vi "Parse Motor Config Data.vi"(7 "Motor NO":u8, 8 "error in (no error)":errorcluster, 10 "PLC Data in":T1, 11 "Data Read":u8[][](array[numeric])) -> (0 "error out":errorcluster, 2 "PLC Data out":T1)   [LabVIEW 2018]
uses:
  Ctls/DisplayIndicator.ctl
  Ctls/MotroConfigData.ctl
  Ctls/MotorConfig.ctl
  Ctls/MagType.ctl
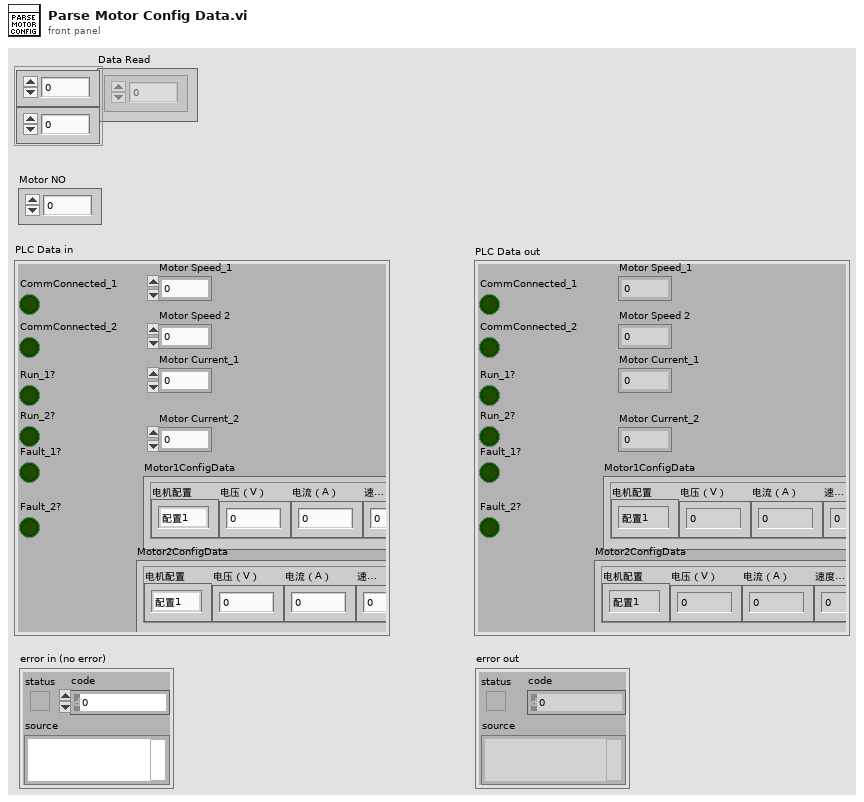
[diagram p1: front panel]
types:
  T1 = typedef "DisplayIndicator.ctl" = cluster{"CommConnected_1":bool, "Run_1?":bool, "Fault_1?":bool, "CommConnected_2":bool, "Run_2?":bool, "Fault_2?":bool, "Motor Speed 2":sgl, "Motor Speed_1":sgl, "Motor Current_1":sgl, "Motor Current_2":sgl, "Motor1ConfigData":T2, "Motor2ConfigData":T2}
  T2 = typedef "MotroConfigData.ctl" = cluster{"电机配置":T3, "电压（V）":dbl, "电流（A）":dbl, "速度（RPM）":dbl, "励磁方式":T4}
  T3 = typedef "MotorConfig.ctl" = enum16{"配置1", "配置2", "配置3", "配置4"}
  T4 = typedef "MagType.ctl" = enum16{"永磁", "励磁"}
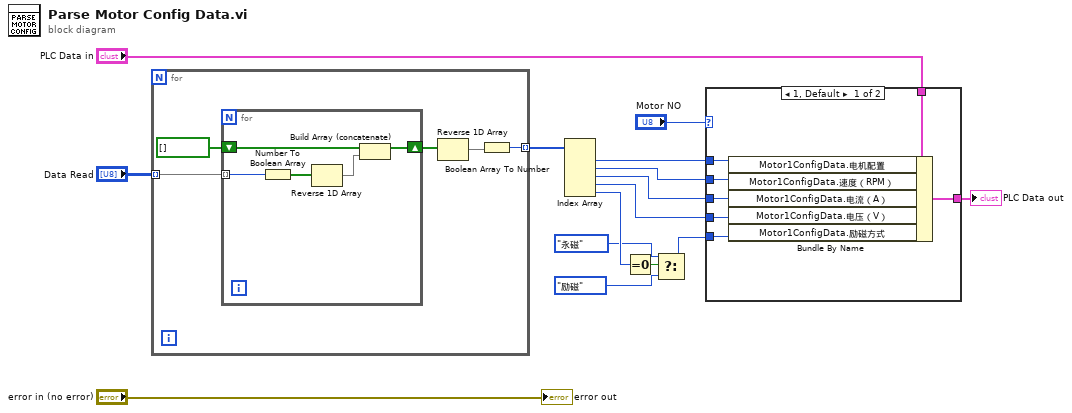
[diagram p0: block diagram]
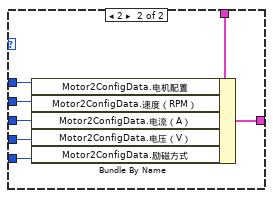
[diagram p2: hidden frame]
diagram:
  n1 = for {
    tunnel: "Data Read" -> [w20] mode=indexing
    tunnel: [w16] -> w11 mode=indexing
    n2 = for {
      tunnel: w20 -> [w25] mode=indexing
      shift-right: [w23] -> w18
      shift-left: bool[] [] ("Boolean array") -> [w24]
      n3 = Number To Boolean Array(number=w25) -> (Boolean array=w22:bool[])
      n4 = Reverse 1D Array(array=w22) -> (reversed array=w21:bool[])
      n5 = Build Array (concatenate)(w24, w21) -> (w23:bool[])
    }
    n6 = Reverse 1D Array(array=w18) -> (reversed array=w17:bool[])
    n7 = Boolean Array To Number(Boolean array=w17) -> (number=w16:u32)
  }
  n8 = Index Array(array=w11) -> (element #1=w10:u32, element #2=w9:u32, element #3=w8:u32, element #4=w7:u32, element #5=w6:u32)  [unwired: 5 in]
  n9 = Equal To 0?(x=w6) -> (x = 0?=w5:bool)
  n10 = Select(t=MagType."永磁" ("Motor1ConfigData.励磁方式"), s=w5, f=MagType."励磁" ("Motor1ConfigData.励磁方式")) -> (s? t:f=w2:T4)
  n11 = case shown="1, Default" "Motor NO" {
    tunnel: "PLC Data in" -> [w32 w39]
    tunnel: [w31 w38] -> w13
    tunnel: w10 -> [w30 w37]
    tunnel: w9 -> [w29 w36]
    tunnel: w8 -> [w28 w35]
    tunnel: w7 -> [w27 w34]
    tunnel: w2 -> [w26 w33]
    frame 1, Default {
      n12 = Bundle By Name(cluster=w32, "Motor1ConfigData.电机配置"=w30, "Motor1ConfigData.速度（RPM）"=w29, "Motor1ConfigData.电流（A）"=w28, "Motor1ConfigData.电压（V）"=w27, "Motor1ConfigData.励磁方式"=w26) -> (w31:T1)
    }
    frame 2 {
      n13 = Bundle By Name(cluster=w39, "Motor2ConfigData.电机配置"=w37, "Motor2ConfigData.速度（RPM）"=w36, "Motor2ConfigData.电流（A）"=w35, "Motor2ConfigData.电压（V）"=w34, "Motor2ConfigData.励磁方式"=w33) -> (w38:T1)
    }
  }
  "PLC Data out" <- w13
  "error out" <- "error in (no error)"
